vi "Write File Header.vi"(4 "Curve Name":string, 5 "App Name":string, 6 "error in":errorcluster, 7 "Hz":dbl format="%.2f", 8 "Control Mode":i32, 9 "File Refnum In":refnum<file>) -> (0 "error out":errorcluster, 3 "File Refnum Out":refnum<file>)   [LabVIEW 2016]
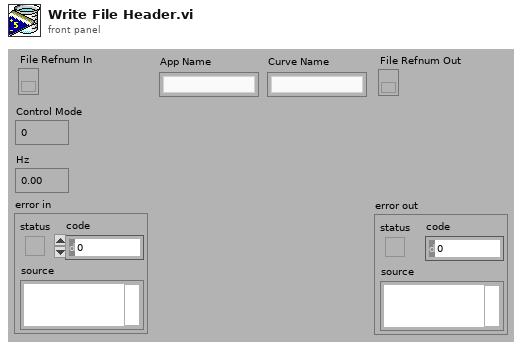
[diagram p1: front panel]
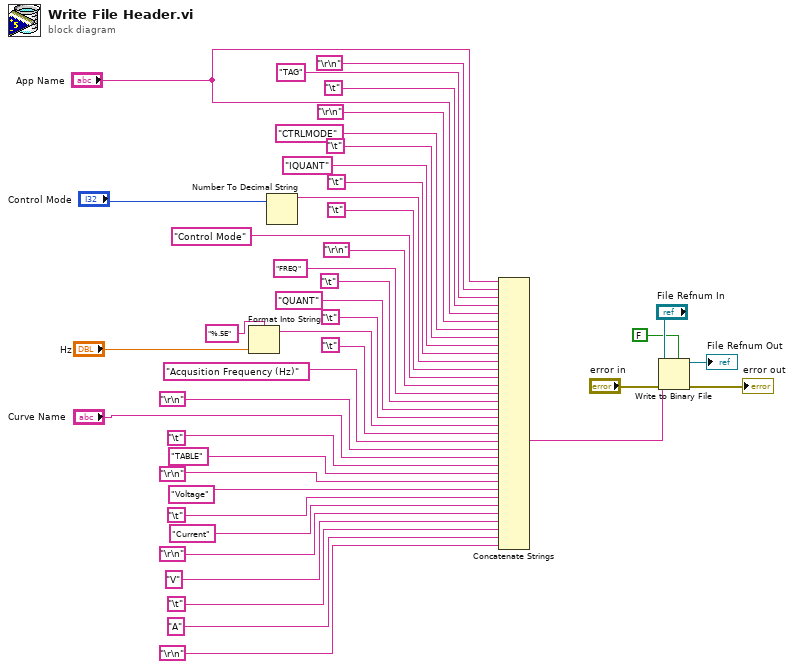
[diagram p0: block diagram]
diagram:
  n1 = Format Into String(format string="%.5E" ("Format String"), "Hz") -> (resulting string=w8:string)  [unwired: 2 in, 1 out]
  n2 = Number To Decimal String(number="Control Mode") -> (decimal integer string=w17:string)  [unwired: 1 in]
  n3 = Concatenate Strings("App Name", "\r\n", "TAG", "\t", "App Name", "\r\n", "CTRLMODE", "\t", "IQUANT", "\t", w17, "\t", "Control Mode", "\r\n", "FREQ", "\t", "QUANT", "\t", w8, "\t", "Acqusition Frequency (Hz)", "\r\n", "Curve Name", "\t", "TABLE", "\r\n", "Voltage", "\t", "Current", "\r\n", "V", "\t", "A", "\r\n") -> (w40:string)
  n4 = Write to Binary File(file (use dialog)="File Refnum In", data=w40, error in="error in", 5:FALSE ("prepend array or string size? (T)")) -> (refnum out=→"File Refnum Out":refnum<file>, error out=→"error out":errorcluster)  [unwired: 2 in, 1 out]
